vi "setGrating.vi"(8 "error in (no error)":errorcluster, 9 "Monochromator in":refnum<class "Monochromator.lvclass">, 10 "GratingType":T1=enum."Red", 11 "SettingUpState in":refnum<class "SettingUpState.lvclass">) -> (0 "error out":errorcluster, 1 "Monochromator out":refnum<class "Monochromator.lvclass">, 3 "SettingUpState out":refnum<class "SettingUpState.lvclass">)   [LabVIEW 2016, in "SettingUpState.lvclass"]
uses:
  SettingUpState.lvclass
  Typedefs/GratingType.ctl
  Monochromator/Monochromator.lvclass
  Typedefs/AckType.ctl
  Monochromator/Monochromator.lvclass/Monochromator.ctl
  MonoCommunicator/MonoCommunicator.lvclass
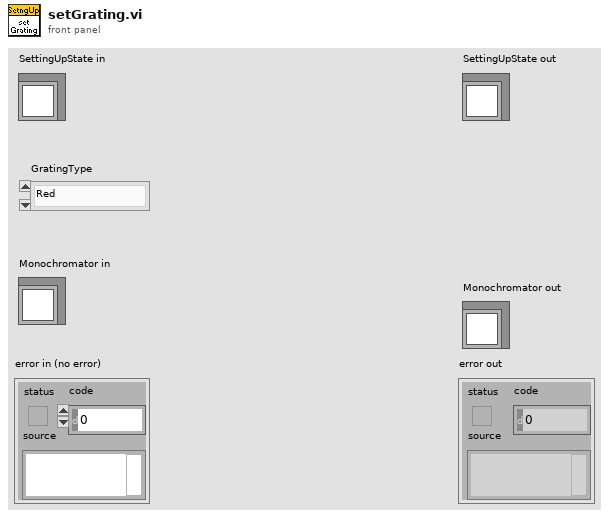
[diagram p1: front panel]
types:
  T1 = typedef "GratingType.ctl" = enum16{"NoGrating", "Red", "Blue", "Mirror"}
  T2 = typedef "AckType.ctl" = enum16{"OK", "OutOfRange", "Unknown", "Busy", "Rejected"}
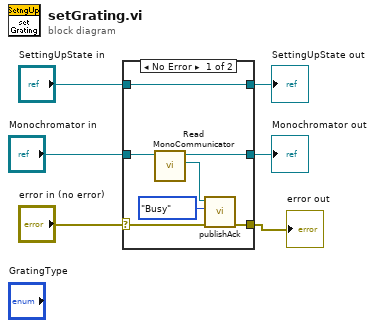
[diagram p0: block diagram]
diagram:
  n1 = case shown="No Error" "error in (no error)" {
    selector: "error in (no error)" -> [w9 w16]
    tunnel: [w8 w16] -> w1
    tunnel: [w13 w15] -> w2
    tunnel: "SettingUpState in" -> [w13 w15]
    tunnel: "Monochromator in" -> [w12 w14]
    tunnel: [w7 w14] -> w3
    frame No Error {
      n2 = call "Read MonoCommunicator.vi"("Monochromator in"=w12) -> ("MonoCommunicator.lvclass"=w11:refnum<class "MonoCommunicator.lvclass">, "Monochromator out"=w7:refnum<class "Monochromator.lvclass">)  [unwired: 8 in, 1 out]
      n3 = call "publishAck.vi"("error in (no error)"=w9, "AckType"=AckType."Busy", "MonoCommunicator in"=w11) -> ("error out"=w8:errorcluster)  [unwired: 7 in, 1 out]
    }
    frame Error {
    }
  }
  "error out" <- w1
  "SettingUpState out" <- w2
  "Monochromator out" <- w3
